vi "AutoCAD NET test.vi"() -> ()   [LabVIEW 2011, in "Design Server.lvlib"]
uses:
  Design Server.lvlib
  C:/Program Files/Autodesk/AutoCAD 2013/Autodesk.AutoCAD.Interop.dll
  Program Files/Autodesk/AutoCAD 2013/Autodesk.AutoCAD.Interop.dll
panel:
  out "new reference":refnum<k24>
  out "doc count error":errorcluster
  out "Version":string
  in  "error in (no error)":errorcluster
  out "error out":errorcluster
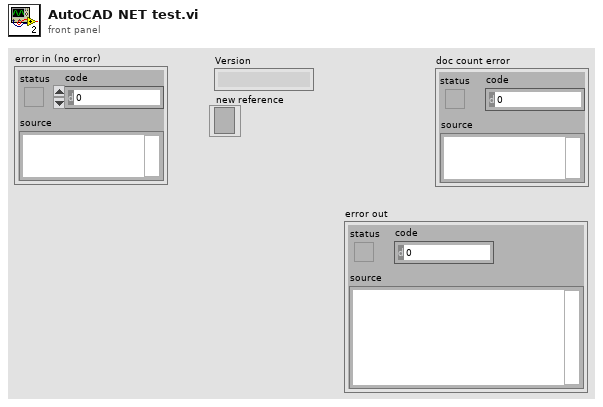
[diagram p1: front panel]
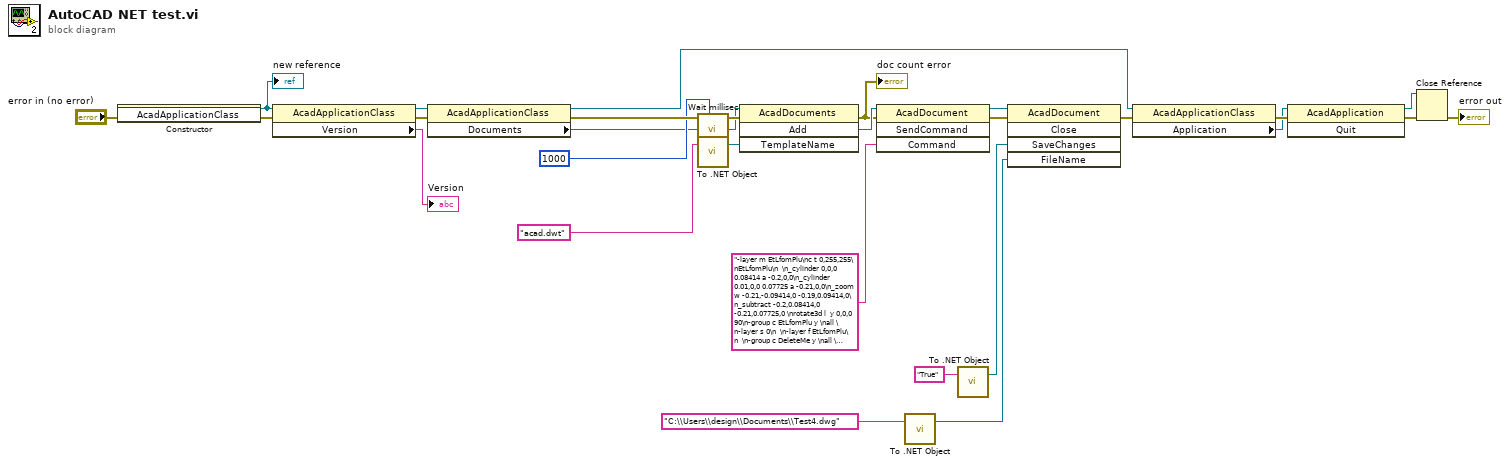
[diagram p0: block diagram]
diagram:
  n1 = constructor class="AcadApplicationClass"(error in="error in (no error)") -> (reference out=w18:refnum<k24>, error out=w8:errorcluster)  [unwired: 2 in, 1 out]
  "new reference" <- w18
  n2 = property class="AcadApplicationClass"(reference=w18, error in=w8) -> (reference out=w16:refnum<k24>, error out=w15:errorcluster, "Version"=→"Version":string)
  n3 = property class="AcadApplicationClass"(reference=w16, error in=w15) -> (reference out=w14:refnum<k24>, error out=w4:errorcluster, "Documents"=w1:refnum<k24>)
  n4 = call "Wait millisec.vi"("milliseconds to wait"=u32 1000, "error in (no error)"=w4) -> ("error out"=w2:errorcluster)  [unwired: 9 in]
  n5 = call <vilib>:"To .NET Object.vi"("anything"="acad.dwt") -> (".NET object"=w7:refnum<k24>)  [unwired: 1 in, 1 out]
  n6 = invoke class="AcadDocuments" method="Add"(reference=w1, error in=w2, "TemplateName"=w7) -> (error out=w5:errorcluster, "Add"=w6:refnum<k24>)  [unwired: 1 in, 2 out]
  "doc count error" <- w5
  n7 = invoke class="AcadDocument" method="SendCommand"(reference=w6, error in=w5, "Command"="-layer m EtLfomPlu\nc t 0,255,255\nEtLfomPlu\n  \n_cylinder 0,0,0 0.08414 a -0.2,0,0\n_cylinder 0.01,0,0 0.07725 a -0.21,0,0\n_zoom w -0.21,-0.09414,0 -0.19,0.09414,0\n_subtract -0.2,0.08414,0  -0.21,0.07725,0 \nrotate3d l  y 0,0,0 90\n-group c EtLfomPlu y \nall \n-layer s 0\n  \n-layer f EtLfomPlu\n  \n-group c DeleteMe y \nall \n-layer t EtLfomPlu\n  \n_subtract\ng EtLfomPlu\n g DeleteMe \n-layer f EtLfomPlu\n  \n-layer t EtLfomPlu\n  \n-layer s EtLfomPlu\n  \n-group c EtLfomPlu y \nall \n-layer s 0\n  \n-layer f EtLfomPlu\n  \n_zoom w -0.01953,-0.01953,-0.09461 0.01953,0.01953,0.01953\n_cylinder 0,0,0.00952 0.00952 a -0.09414,0,0.00952\nrotate3d l  z 0,0,0.00952 97.3515\n-array l  P 0,0,0.00952 8 114.84123 Y\n_zoom w -0.01953,-0.01953,-0.07461 0.01953,0.01953,0.03952\n_cylinder 0,0,0.02953 0.00952 a -0.09414,0,0.02953\nrotate3d l  z 0,0,0.02953 90\n_zoom w -0.01953,-0.01953,-0.05461 0.01953,0.01953,0.05953\n_cylinder 0,0,0.04953 0.00952 a -0.09414,0,0.04953\nrotate3d l  z 0,0,0.04953 97.3515\n-array l  P 0,0,0.04953 3 32.81178 Y\n_zoom w -0.01953,-0.01953,-0.03461 0.01953,0.01953,0.07953\n_cylinder 0,0,0.06953 0.00952 a -0.09414,0,0.06953\nrotate3d l  z 0,0,0.06953 90\n-array l  P 0,0,0.06953 2 16.40589 Y\n_zoom w -0.01953,-0.01953,-0.01461 0.01953,0.01953,0.09952\n_cylinder 0,0,0.08953 0.00952 a -0.09414,0,0.08953\nrotate3d l  z 0,0,0.08953 97.3515\n_zoom w -0.01953,-0.01953,0.00539 0.01953,0.01953,0.11953\n_cylinder 0,0,0.10953 0.00952 a -0.09414,0,0.10953\nrotate3d l  z 0,0,0.10953 90\n-array l  P 0,0,0.10953 2 16.40589 Y\n_zoom w -0.01953,-0.01953,0.02539 0.01953,0.01953,0.13953\n_cylinder 0,0,0.12953 0.00952 a -0.09414,0,0.12953\nrotate3d l  z 0,0,0.12953 97.3515\n_zoom w -0.01953,-0.01953,0.04539 0.01953,0.01953,0.15953\n_cylinder 0,0,0.14953 0.00952 a -0.09414,0,0.14953\nrotate3d l  z 0,0,0.14953 90\n-array l  P 0,0,0.14953 2 16.40589 Y\n_zoom w -0.01953,-0.01953,0.06539 0.01953,0.01953,0.17953\n_cylinder 0,0,0.16953 0.00952 a -0.09414,0,0.16953\nrotate3d l  z 0,0,0.16953 97.3515\n_zoom w -0.01953,-0.01953,0.08539 0.01953,0.01953,0.19953\n_cylinder 0,0,0.18953 0.00952 a -0.09414,0,0.18953\nrotate3d l  z 0,0,0.18953 90\n-group c DeleteMe y \nall \n-layer t EtLfomPlu\n  \n_subtract\ng EtLfomPlu\n g DeleteMe \n-layer f EtLfomPlu\n  \nlaythw\n_-view o f\n-plot y \nPublishToWeb PNG.pc3\nVGA (640.00 x 480.00 Pixels)\nl n e F\n\n .\ny  D:\\inetpub\\wwwroot\\Designs\\LFOM\\5177\\6Lps\\LFOM_f\nn y\nshademode x -view swiso ") -> (reference out=w24:refnum<k24>, error out=w21:errorcluster)  [unwired: 1 in, 2 out]
  n8 = call <vilib>:"To .NET Object.vi"("anything"="C:\\Users\\design\\Documents\\Test4.dwg") -> (".NET object"=w23:refnum<k24>)  [unwired: 1 in, 1 out]
  n9 = call <vilib>:"To .NET Object.vi"("anything"="True") -> (".NET object"=w20:refnum<k24>)  [unwired: 1 in, 1 out]
  n10 = invoke class="AcadDocument" method="Close"(reference=w24, error in=w21, "SaveChanges"=w20, "FileName"=w23) -> (error out=w13:errorcluster)  [unwired: 1 in, 4 out]
  n11 = property class="AcadApplicationClass"(reference=w14, error in=w13) -> (error out=w12:errorcluster, "Application"=w11:refnum<k24>)  [unwired: 1 out]
  n12 = invoke class="AcadApplication" method="Quit"(reference=w11, error in=w12) -> (reference out=w9:refnum<k24>, error out=w10:errorcluster)  [unwired: 1 in, 1 out]
  n13 = Close Reference(reference=w9, error in (no error)=w10) -> (error out=→"error out":errorcluster)
